vi "Read OOI List.vi"() -> (2 "ObjectsOfInterest":T1(array[cluster]))   [LabVIEW 2014]
uses:
  <vilib>/xml/Load XML File.vi
  <resource>/objmgr/DOMUserDefRef.rc
  <vilib>/xml/NI_XML.lvlib
panel:
  out "appended path":path
  in  "error in (no error)":errorcluster
  out "error out":errorcluster
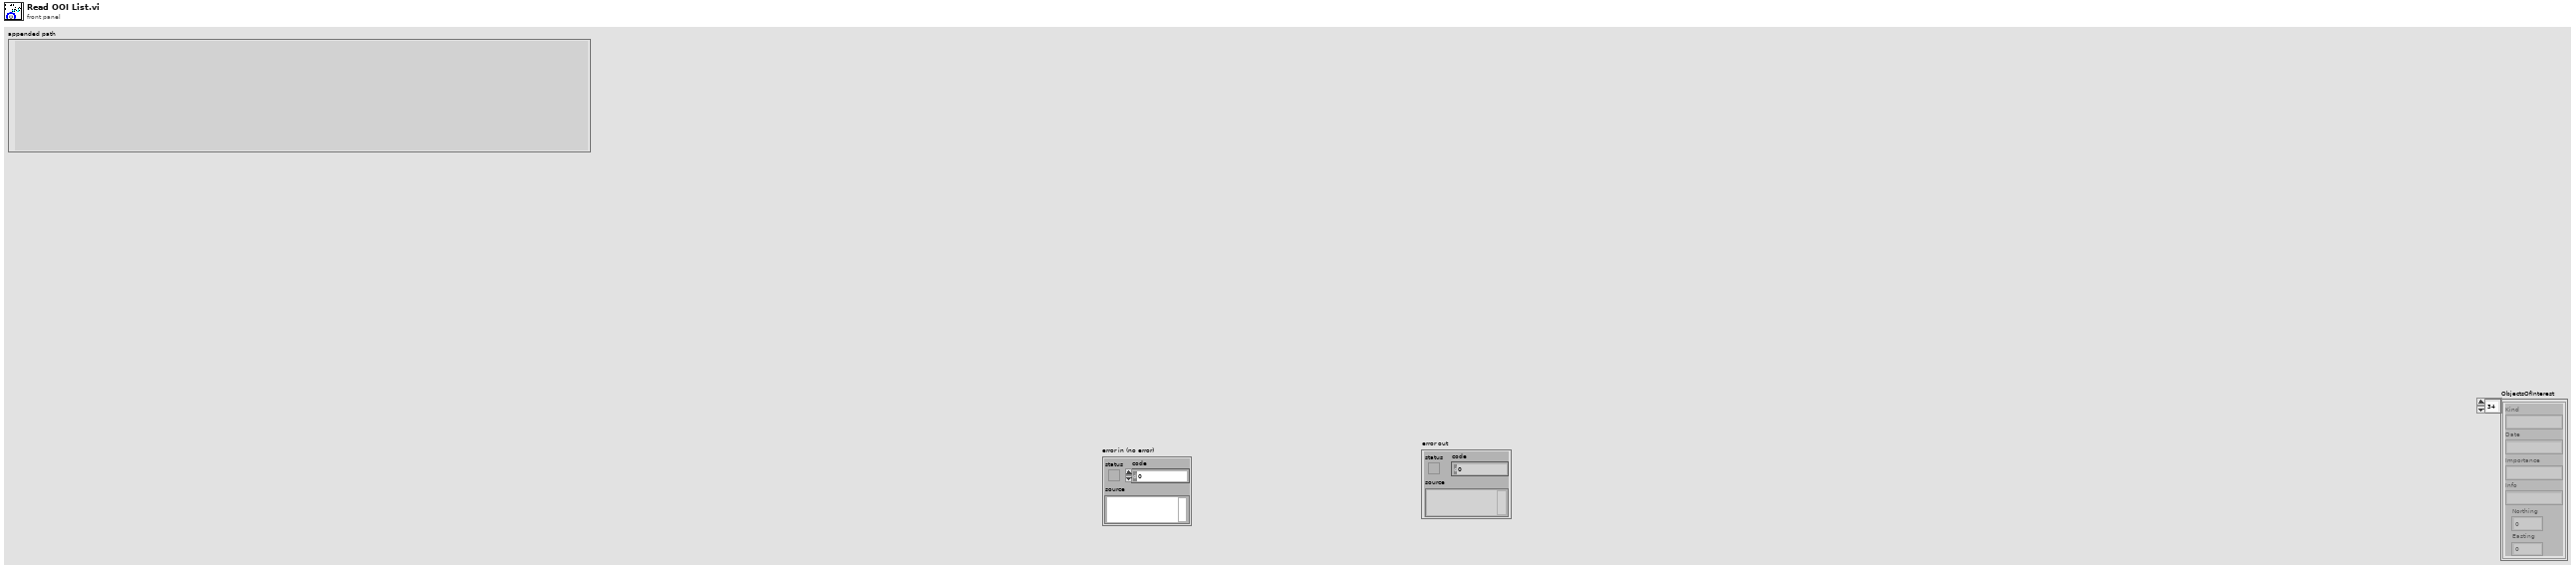
[diagram p1: front panel]
types:
  T1 = cluster{"Kind":string, "Date":string, "Importance":string, "Info":string, "Northing":dbl, "Easting":dbl}[]
  T2 = cluster{"Kind":string, "Date":string, "Importance":string, "Info":string, "Northing":dbl, "Easting":dbl}
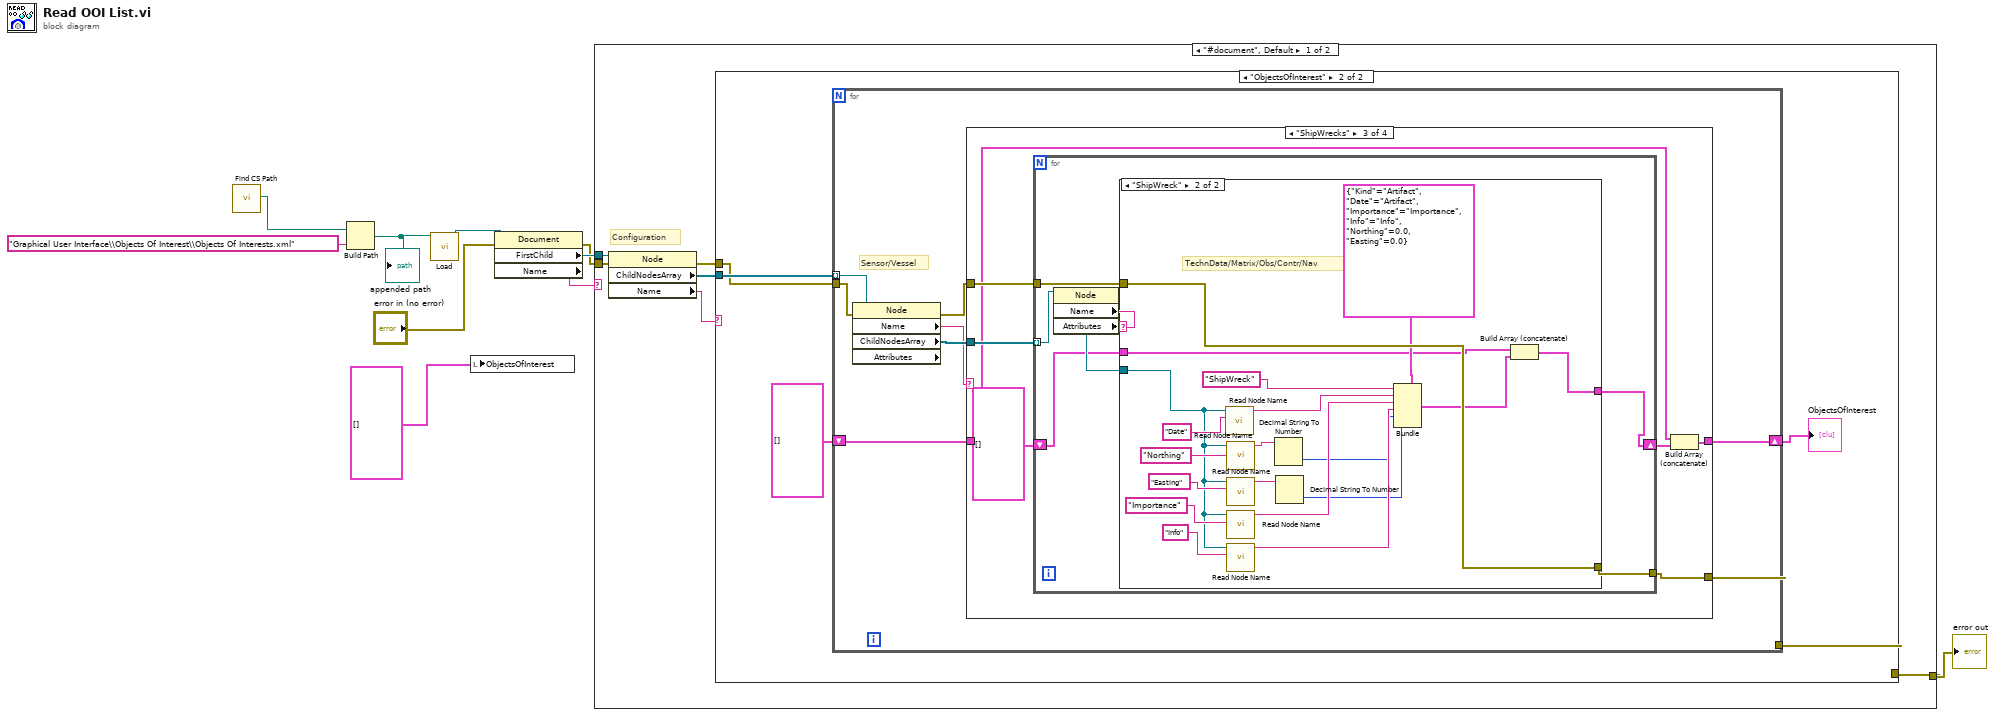
[diagram p0: block diagram]
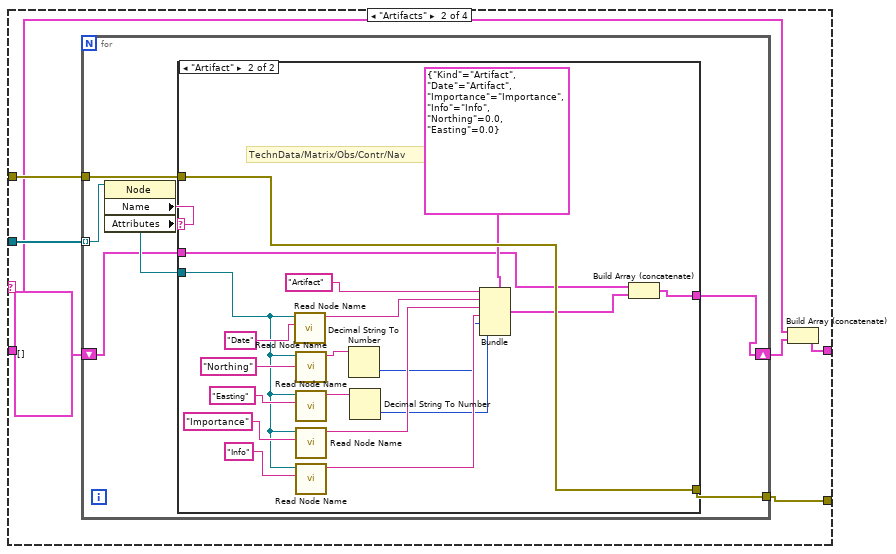
[diagram p4: hidden frame]
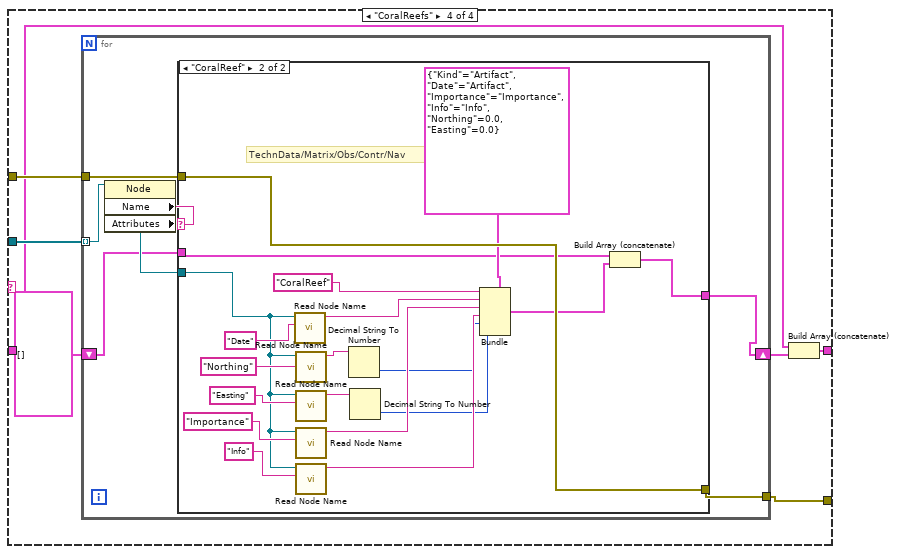
[diagram p7: hidden frame]
diagram:
  n1 = call "Find CS Path.vi"() -> ("path to CS folder"=w2:path)  [unwired: 11 in]
  n2 = Build Path(base path=w2, name or relative path="Graphical User Interface\\Objects Of Interest\\Objects Of Interests.xml") -> (appended path=w3:path)
  "appended path" <- w3
  n3 = call-poly <vilib>:"Load.vi"("path to XML document"=w3) -> ("DOM document out"=w10:refnum<k20>)  [unwired: 12 in, 2 out]
  n4 = local write "ObjectsOfInterest"(T1 []) -> ()
  n5 = property class="Document"(reference=w10, error in="error in (no error)") -> (error out=w7:errorcluster, "FirstChild"=w9:refnum<k20>, "Name"=w8:string)  [unwired: 1 out]
  n6 = case shown="\"#document\", Default" w8 {
    tunnel: w9 -> [w16 _]
    tunnel: w7 -> [w13 w138]
    tunnel: [w11 w138] -> w5
    frame "#document", Default {
      # "Configuration"
      n7 = property class="Node"(reference=w16, error in=w13) -> (error out=w12:errorcluster, "ChildNodesArray"=w14:refnum<k20>[], "Name"=w15:string)  [unwired: 1 out]
      n8 = case shown="\"ObjectsOfInterest\"" w15 {
        tunnel: w14 -> [_ w22]
        tunnel: w12 -> [w17 w21]
        tunnel: [w17 w20] -> w11
        frame "#~", Default {
        }
        frame "ObjectsOfInterest" {
          n9 = for {
            tunnel: w22 -> [w30] mode=indexing
            tunnel: w21 -> [w28]
            tunnel: [w26] -> w20
            shift-right: [w24] -> w19
            shift-left: T1 [] -> [w23]
            # "Sensor/Vessel"
            n10 = property class="Node" props=["Name", "ChildNodesArray", "Attributes"](reference=w30, error in=w28) -> (error out=w27:errorcluster, "Name"=w25:string, "ChildNodesArray"=w29:refnum<k20>[])  [unwired: 2 out]
            n11 = case shown="\"ShipWrecks\"" w25 {
              tunnel: w29 -> [_ w37 w72 w107]
              tunnel: w27 -> [w32 w39 w74 w109]
              tunnel: [w32 w38 w73 w108] -> w26
              tunnel: [w31 w33 w68 w104] -> w24
              tunnel: w23 -> [w31 w35 w69 w103]
              frame "#~", Default {
              }
              frame "Artifacts" {
                n12 = for {
                  tunnel: w37 -> [w44] mode=indexing
                  tunnel: w39 -> [w46]
                  tunnel: [w45] -> w38
                  shift-right: [w40] -> w34
                  shift-left: T1 [] -> [w41]
                  n13 = property class="Node"(reference=w44) -> ("Name"=w43:string, "Attributes"=w42:refnum<k20>)  [unwired: 1 in, 2 out]
                  n14 = case shown="\"Artifact\"" w43 {
                    tunnel: w46 -> [w48 w67]
                    tunnel: [w48 w67] -> w45
                    tunnel: w42 -> [_ w61]
                    tunnel: w41 -> [w47 w50]
                    tunnel: [w47 w49] -> w40
                    frame "#~", Default {
                    }
                    frame "Artifact" {
                      # "TechnData/Matrix/Obs/Contr/Nav"
                      n15 = call "Read Node Name.vi"("Name"="Date", "Attributes"=w61) -> ("Value"=w57:string)  [unwired: 9 in]
                      n16 = call "Read Node Name.vi"("Name"="Northing", "Attributes"=w61) -> ("Value"=w54:string)  [unwired: 9 in]
                      n17 = call "Read Node Name.vi"("Name"="Easting", "Attributes"=w61) -> ("Value"=w55:string)  [unwired: 9 in]
                      n18 = call "Read Node Name.vi"("Name"="Importance", "Attributes"=w61) -> ("Value"=w58:string)  [unwired: 9 in]
                      n19 = call "Read Node Name.vi"("Name"="Info", "Attributes"=w61) -> ("Value"=w59:string)  [unwired: 9 in]
                      n20 = Decimal String To Number(string=w54) -> (number=w52:i32)  [unwired: 2 in, 1 out]
                      n21 = Decimal String To Number(string=w55) -> (number=w53:i32)  [unwired: 2 in, 1 out]
                      n22 = Bundle(cluster=T2 {"Kind"="Artifact", "Date"="Artifact", "Importance"="Importance", "Info"="Info", "Northing"=0.0, "Easting"=0.0}, "Kind"="Artifact" ("Name"), "Date"=w57, "Importance"=w58, "Info"=w59, "Northing"=w52, "Easting"=w53) -> (w51:T2)
                      n23 = Build Array (concatenate)(w50, w51) -> (w49:T1)
                    }
                  }
                }
                n24 = Build Array (concatenate)(w35, w34) -> (w33:T1)
              }
              frame "ShipWrecks" {
                n25 = for {
                  tunnel: w72 -> [w79] mode=indexing
                  tunnel: w74 -> [w81]
                  tunnel: [w80] -> w73
                  shift-right: [w75] -> w70
                  shift-left: T1 [] -> [w76]
                  n26 = property class="Node"(reference=w79) -> ("Name"=w78:string, "Attributes"=w77:refnum<k20>)  [unwired: 1 in, 2 out]
                  n27 = case shown="\"ShipWreck\"" w78 {
                    tunnel: w81 -> [w83 w102]
                    tunnel: [w83 w102] -> w80
                    tunnel: w77 -> [_ w96]
                    tunnel: w76 -> [w82 w84]
                    tunnel: [w82 w86] -> w75
                    frame "#~", Default {
                    }
                    frame "ShipWreck" {
                      # "TechnData/Matrix/Obs/Contr/Nav"
                      n28 = call "Read Node Name.vi"("Name"="Date", "Attributes"=w96) -> ("Value"=w92:string)  [unwired: 9 in]
                      n29 = call "Read Node Name.vi"("Name"="Northing", "Attributes"=w96) -> ("Value"=w89:string)  [unwired: 9 in]
                      n30 = call "Read Node Name.vi"("Name"="Easting", "Attributes"=w96) -> ("Value"=w90:string)  [unwired: 9 in]
                      n31 = call "Read Node Name.vi"("Name"="Importance", "Attributes"=w96) -> ("Value"=w93:string)  [unwired: 9 in]
                      n32 = call "Read Node Name.vi"("Name"="Info", "Attributes"=w96) -> ("Value"=w94:string)  [unwired: 9 in]
                      n33 = Decimal String To Number(string=w89) -> (number=w87:i32)  [unwired: 2 in, 1 out]
                      n34 = Decimal String To Number(string=w90) -> (number=w88:i32)  [unwired: 2 in, 1 out]
                      n35 = Bundle(cluster=T2 {"Kind"="Artifact", "Date"="Artifact", "Importance"="Importance", "Info"="Info", "Northing"=0.0, "Easting"=0.0}, "Kind"="ShipWreck" ("Name"), "Date"=w92, "Importance"=w93, "Info"=w94, "Northing"=w87, "Easting"=w88) -> (w85:T2)
                      n36 = Build Array (concatenate)(w84, w85) -> (w86:T1)
                    }
                  }
                }
                n37 = Build Array (concatenate)(w69, w70) -> (w68:T1)
              }
              frame "CoralReefs" {
                n38 = for {
                  tunnel: w107 -> [w114] mode=indexing
                  tunnel: w109 -> [w116]
                  tunnel: [w115] -> w108
                  shift-right: [w110] -> w105
                  shift-left: T1 [] -> [w111]
                  n39 = property class="Node"(reference=w114) -> ("Name"=w113:string, "Attributes"=w112:refnum<k20>)  [unwired: 1 in, 2 out]
                  n40 = case shown="\"CoralReef\"" w113 {
                    tunnel: w116 -> [w118 w137]
                    tunnel: [w118 w137] -> w115
                    tunnel: w112 -> [_ w131]
                    tunnel: w111 -> [w117 w120]
                    tunnel: [w117 w121] -> w110
                    frame "#~", Default {
                    }
                    frame "CoralReef" {
                      # "TechnData/Matrix/Obs/Contr/Nav"
                      n41 = call "Read Node Name.vi"("Name"="Date", "Attributes"=w131) -> ("Value"=w127:string)  [unwired: 9 in]
                      n42 = call "Read Node Name.vi"("Name"="Northing", "Attributes"=w131) -> ("Value"=w124:string)  [unwired: 9 in]
                      n43 = call "Read Node Name.vi"("Name"="Easting", "Attributes"=w131) -> ("Value"=w125:string)  [unwired: 9 in]
                      n44 = call "Read Node Name.vi"("Name"="Importance", "Attributes"=w131) -> ("Value"=w128:string)  [unwired: 9 in]
                      n45 = call "Read Node Name.vi"("Name"="Info", "Attributes"=w131) -> ("Value"=w129:string)  [unwired: 9 in]
                      n46 = Decimal String To Number(string=w124) -> (number=w122:i32)  [unwired: 2 in, 1 out]
                      n47 = Decimal String To Number(string=w125) -> (number=w123:i32)  [unwired: 2 in, 1 out]
                      n48 = Bundle(cluster=T2 {"Kind"="Artifact", "Date"="Artifact", "Importance"="Importance", "Info"="Info", "Northing"=0.0, "Easting"=0.0}, "Kind"="CoralReef" ("Name"), "Date"=w127, "Importance"=w128, "Info"=w129, "Northing"=w122, "Easting"=w123) -> (w119:T2)
                      n49 = Build Array (concatenate)(w120, w119) -> (w121:T1)
                    }
                  }
                }
                n50 = Build Array (concatenate)(w103, w105) -> (w104:T1)
              }
            }
          }
          "ObjectsOfInterest" <- w19
        }
      }
    }
    frame "~" {
    }
  }
  "error out" <- w5
